vi "Direttore.fpga.vi"   [LabVIEW 2012]
uses:
  <vilib>/rvi/interface/RandomDataEmulation/nirviRandomDataFPGAFIFO.vi
  <vilib>/rvi/interface/RandomDataEmulation/niFpgaRandomDataHandleErrors.vi
  <vilib>/rvi/DataTransferAndStorage/Container/XNode/niFpgaContainer.xnode
  <vilib>/rvi/interface/RandomDataEmulation/nirviRandomDataFpgaReadWriteTemplate.vi
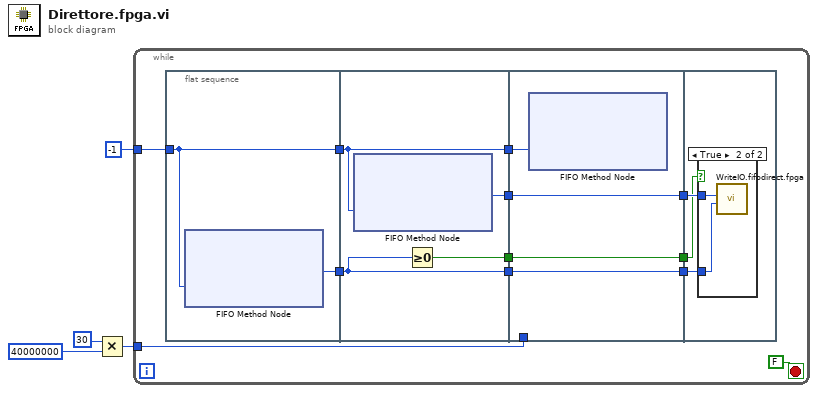
[diagram p0: block diagram]
diagram:
  n1 = Multiply(x=u32 30, y=u32 40000000) -> (x*y=w1:u32)
  n2 = while {
    tunnel: -1 ("Timeout") -> [w14]
    tunnel: w1 -> [w6]
    stop <- FALSE stop-if-true
    n3 = flat-sequence {
      tunnel: w14 -> [w18]
      tunnel: [w18] -> w12
      tunnel: [w17] -> w10
      tunnel: [w21] -> w13
      tunnel: w12 -> [w22]
      tunnel: [w22] -> w11
      tunnel: w10 -> [w19]
      tunnel: [w19] -> w9
      tunnel: [w20] -> w8
      tunnel: [w23] -> w16
      tunnel: [w25] -> w15
      tunnel: w13 -> [w23]
      tunnel: w11 -> [w26]
      tunnel: w9 -> [w25]
      tunnel: w8 -> [w24]
      tunnel: [w24] -> w7
      tunnel: w6 -> [_]
      tunnel: w16 -> [w28]
      tunnel: w15 -> [w29]
      tunnel: w7 -> [w27]
      frame #0 {
        n4 = xnode ("FIFO Method Node")("Timeout"=w18) -> ("Element"=w17:i32)  [unwired: 1 in, 2 out]
      }
      frame #1 {
        n5 = xnode ("FIFO Method Node")("Timeout"=w22) -> ("Element"=w21:i32)  [unwired: 1 in, 2 out]
        n6 = Greater Or Equal To 0?(x=w19) -> (x >= 0?=w20:bool)
      }
      frame #2 {
        n7 = xnode ("FIFO Method Node")("Timeout"=w26) -> ()  [unwired: 1 in, 3 out]
      }
      frame #3 {
        n8 = case shown="True" w27 {
          tunnel: w28 -> [_ w30]
          tunnel: w29 -> [_ w31]
          frame False {
          }
          frame True {
            n9 = call "WriteIO.fifodirect.fpga.vi"("Delta time"=w31, "Number of time points"=w30) -> ()  [unwired: 10 in]
          }
        }
      }
    }
  }
